vi "Write Stop Rendezvous.vi"(8 "error in (no error)":errorcluster, 10 "rendezvous":T1, 11 "bt_System in":refnum<class "bt_System.lvclass">) -> (0 "error out":errorcluster, 3 "bt_System out":refnum<class "bt_System.lvclass">)   [LabVIEW 2021, in "BT.lvlib" / "bt_System.lvclass"]
uses:
  bt_System.lvclass
  bt_System.lvclass/bt_System.ctl
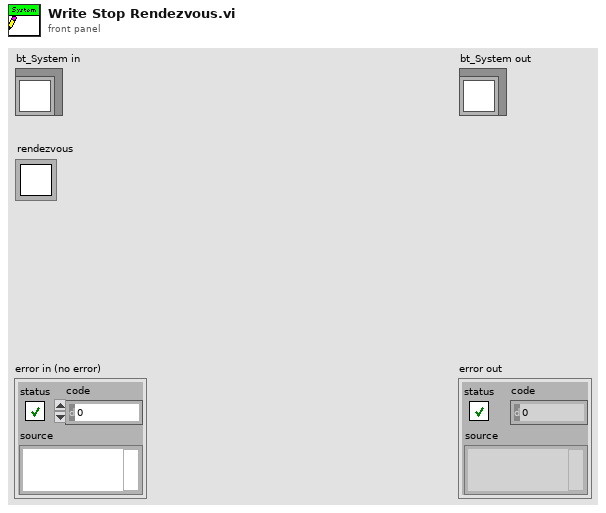
[diagram p1: front panel]
types:
  T1 = typedef "Rendezvous RefNum" = refnum<k1>
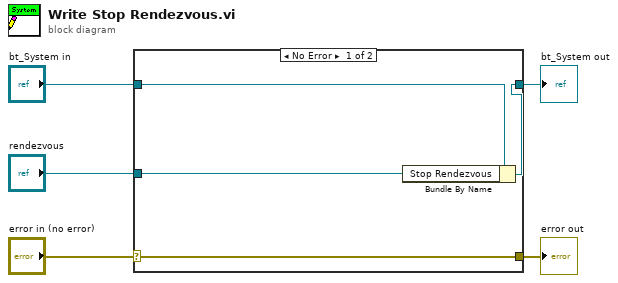
[diagram p0: block diagram]
diagram:
  n1 = case shown="No Error" "error in (no error)" {
    selector: "error in (no error)" -> [w9 w10]
    tunnel: [w9 w10] -> w4
    tunnel: [w7 w11] -> w2
    tunnel: "bt_System in" -> [w8 w11]
    tunnel: "rendezvous" -> [w6 _]
    frame No Error {
      n2 = Bundle By Name(cluster=w8, "Stop Rendezvous"=w6) -> (w7:refnum<class "bt_System.lvclass">)
    }
    frame Error {
    }
  }
  "error out" <- w4
  "bt_System out" <- w2
